vi "Play_Init.vi"(0 "object in":refnum<class "Play.lvclass">, 2 "number_of_robots":i32, 5 "error in (no error)":errorcluster) -> (14 "object out":refnum<class "Play.lvclass">, 19 "error out":errorcluster)   [LabVIEW 2023, in "Play.lvclass"]
uses:
  Play.lvclass
  Play.lvclass/Play.ctl
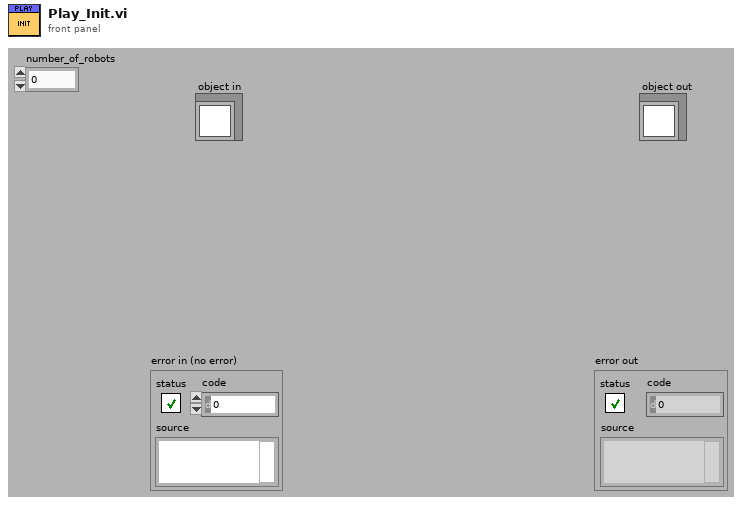
[diagram p1: front panel]
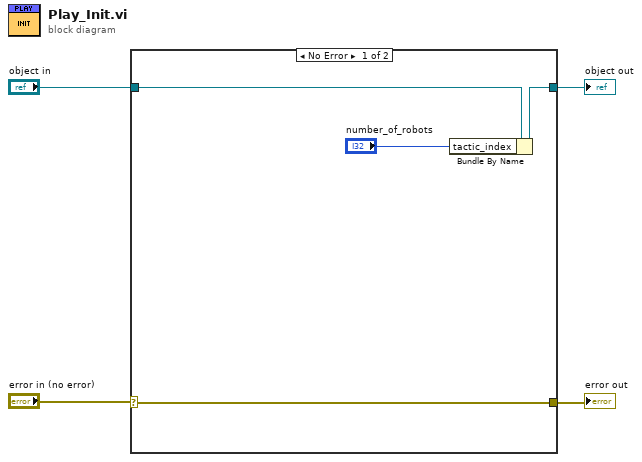
[diagram p0: block diagram]
diagram:
  n1 = case shown="No Error" "error in (no error)" {
    selector: "error in (no error)" -> [w6 w9]
    tunnel: "object in" -> [w8 w10]
    tunnel: [w7 w10] -> w3
    tunnel: [w6 w9] -> w1
    frame No Error {
      n2 = Bundle By Name(cluster=w8, "tactic_index"="number_of_robots") -> (w7:refnum<class "Play.lvclass">)
    }
    frame Error {
    }
  }
  "object out" <- w3
  "error out" <- w1
